vi "UpdateSettings.channelCluster.vi"(8 "error in (no error)":errorcluster, 10 "ChannelName":string, 11 "TektronixDPO in":refnum<class "TektronixDPO.lvclass">) -> (0 "error out":errorcluster, 3 "TektronixDPO out":refnum<class "TektronixDPO.lvclass">)   [LabVIEW 2013, in "TektronixDPO.lvclass"]
doc: "Update the settings cluster"
uses:
  TektronixDPO.lvclass
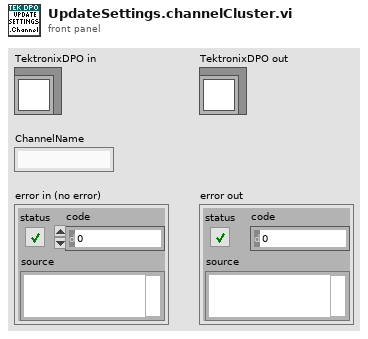
[diagram p1: front panel]
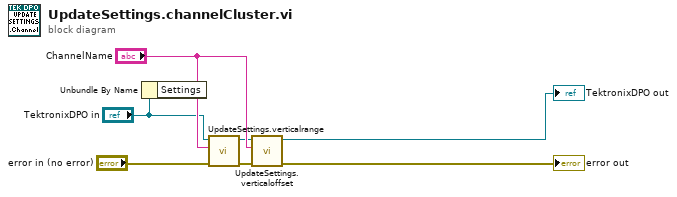
[diagram p0: block diagram]
diagram:
  n1 = Unbundle By Name("TektronixDPO in") -> ()  [unwired: 1 out]
  n2 = call "UpdateSettings.verticalrange.vi"("error in (no error)"="error in (no error)", "ChannelName"="ChannelName", "TektronixDPO in"="TektronixDPO in") -> ("error out"=w5:errorcluster, "TektronixDPO out"=w3:refnum<class "TektronixDPO.lvclass">)  [unwired: 7 in]
  n3 = call "UpdateSettings.verticaloffset.vi"("error in (no error)"=w5, "ChannelName"="ChannelName", "TektronixDPO in"=w3) -> ("error out"=→"error out":errorcluster, "TektronixDPO out"=→"TektronixDPO out":refnum<class "TektronixDPO.lvclass">)  [unwired: 7 in]
